vi "Draw Tree.vi"(10 "Sequencing Data":T1) -> (2 "Tree":T1, 3 "2D Picture":picture)   [LabVIEW 2025]
uses:
  Types/Decision Tree.ctl
  Types/Sequencing Tree Node.ctl
  Types/Single Cmd Info.ctl
  <vilib>/picture/picture.llb/imagedata.ctl
panel:
  in  "Outcome Font":T5={"Font Name:"="Bahnschrift", "Size"=15, "Strikeout?"=FALSE, "Italic?"=FALSE, "Underline?"=TRUE, "Outline?"=FALSE, "Shadow?"=FALSE, "Bold?"=TRUE}
  in  "Height Padding":i32=8
  in  "Leaf + Outcome Name Height":i32=38
  in  "Leaf Width":i32=16
  in  "Command Height":i32=32
  in  "Path on Command Branch Height":i32=35
  in  "Default Path Height":i32=15
  in  "Leaf Height":i32=16
  in  "Leaf Circle Radius":i32=8
  in  "pen":T6={"Width"=3, "Style"=enum."Solid"}
  in  "2D Picture":picture
  in  "Column Gap":i32=30
  in  "[user-specified font]":T5={"Font Name:"="Bahnschrift", "Size"=15, "Strikeout?"=FALSE, "Italic?"=FALSE, "Underline?"=FALSE, "Outline?"=FALSE, "Shadow?"=FALSE, "Bold?"=FALSE}
  in  "Width Padding":i32=8
  in  "Row Gap":i32=40
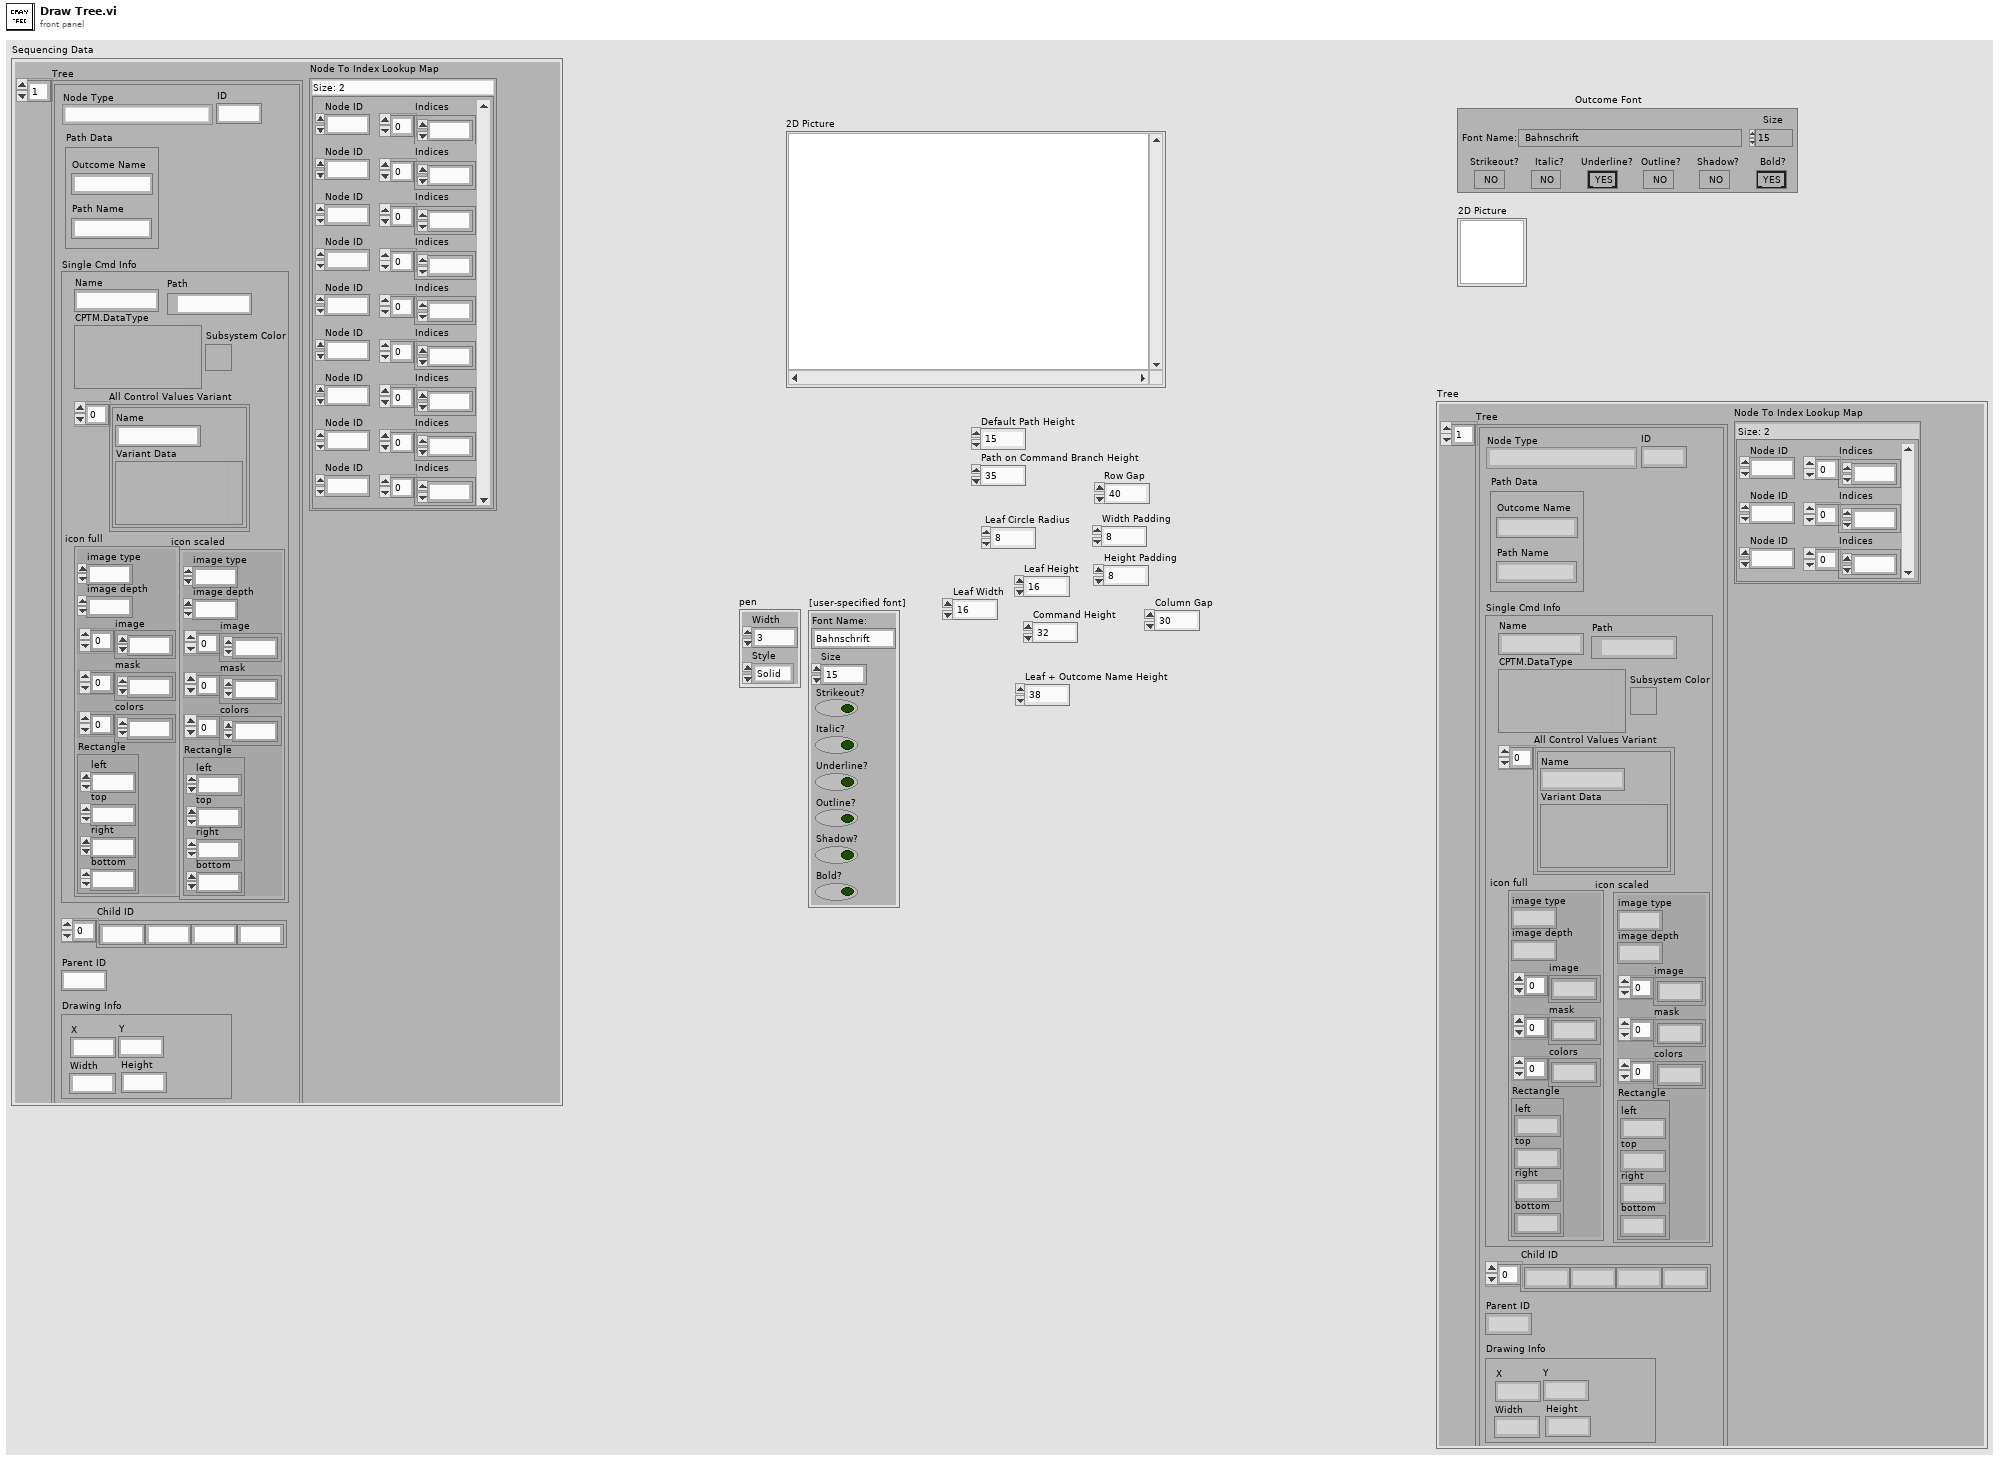
[diagram p1: front panel]
types:
  T1 = typedef "Decision Tree.ctl" = cluster{"Tree":T2[], "Node To Index Lookup Map":map{i16, i16[]}}
  T2 = typedef "Sequencing Tree Node.ctl" = cluster{"Node Type":enum16{"Path", "Command", "Leaf"}, "ID":i16, "Path Data":cluster{"Path Name":string, "Outcome Name":string}, "Single Cmd Info":T3, "Child ID":i32[], "Parent ID":i32, "Drawing Info":cluster{"X":i32, "Y":i32, "Width":i32, "Height":i32}}
  T3 = typedef "Single Cmd Info.ctl" = cluster{"Name":string, "CPTM.DataType":variant, "All Control Values Variant":cluster{"Name":string, "Variant Data":variant}[], "icon full":T4, "icon scaled":T4, "Path":path, "Subsystem Color":u32}
  T4 = typedef "imagedata.ctl" = cluster{"image type":i32, "image depth":i32, "image":u8[], "mask":u8[], "colors":u32[], "Rectangle":cluster{"left":i16, "top":i16, "right":i16, "bottom":i16}}
  T5 = cluster{"Font Name:":string, "Size":i16, "Strikeout?":bool, "Italic?":bool, "Underline?":bool, "Outline?":bool, "Shadow?":bool, "Bold?":bool}
  T6 = cluster{"Width":i16, "Style":enum32{"Solid", "Dash", "Dot", "DashDot", "DashDotDot"}}
  T7 = cluster{"X":i32, "Y":i32, "Width":i32, "Height":i32}
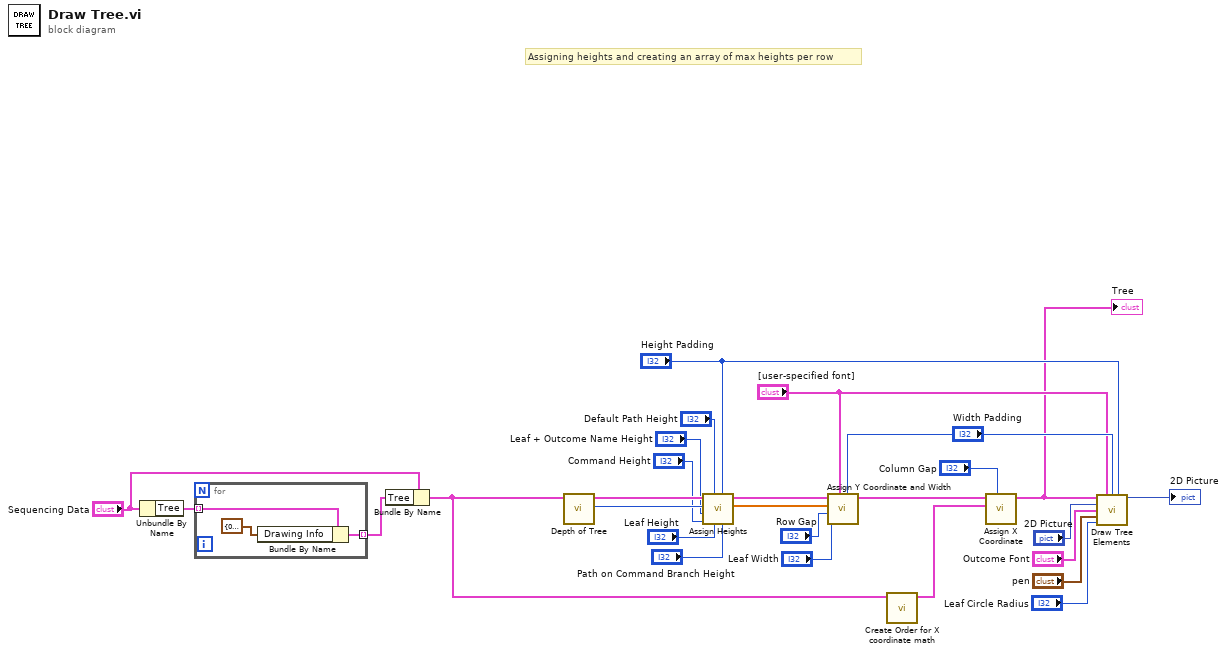
[diagram p0: block diagram]
diagram:
  # "Assigning heights and creating an array of max heights per row"
  n1 = Unbundle By Name("Sequencing Data") -> ("Tree"=w4:T2[])
  n2 = for {
    tunnel: w4 -> [w30] mode=indexing
    tunnel: [w28] -> w3 mode=indexing
    n3 = Bundle By Name(cluster=w30, "Drawing Info"=T7 {"X"=0, "Y"=0, "Width"=0, "Height"=0}) -> (w28:T2)
  }
  n4 = Bundle By Name(cluster="Sequencing Data", "Tree"=w3) -> (w1:T1)
  n5 = call "Depth of Tree.vi"("Tree in"=w1) -> ("Depth"=w24:i32, "Tree with Depths"=w27:T1)  [unwired: 9 in]
  n6 = call "Assign Heights.vi"("Path on Command Branch Height"="Path on Command Branch Height", "Height Padding"="Height Padding", "Leaf Height"="Leaf Height", "Default Path Height"="Default Path Height", "Command Height"="Command Height", "Leaf + Outcome Name Height"="Leaf + Outcome Name Height", "Depth"=w24, "Tree with Depths in"=w27) -> ("Max Height per Row"=w16:dbl[], "Tree with Heights Out"=w17:T1)  [unwired: 2 in]
  n7 = call "Assign Y Coordinate and Width.vi"("Width Padding"="Width Padding", "[user-specified font]"="[user-specified font]", "Leaf Width"="Leaf Width", "Row Gap"="Row Gap", "Max Height per Row"=w16, "Tree with Heights in"=w17) -> ("Decision Tree Out"=w26:T1)  [unwired: 5 in]
  n8 = call "Create Order for X coordinate math.vi"("Tree"=w1) -> ("Array"=w25:T2[])  [unwired: 10 in]
  n9 = call "Assign X Coordinate.vi"("Column Gap"="Column Gap", "Order"=w25, "Decision Tree Out in"=w26) -> ("Decision Tree Out out"=w5:T1)  [unwired: 8 in]
  "Tree" <- w5
  n10 = call "Draw Tree Elements.vi"("Decision Tree In"=w5, "[user-specified font]"="[user-specified font]", "Width Padding"="Width Padding", "Height Padding"="Height Padding", "2D Picture in"="2D Picture", "Outcome Font"="Outcome Font", "pen"="pen", "Leaf Circle Radius"="Leaf Circle Radius") -> ("2D Picture out"=→"2D Picture":picture)  [unwired: 7 in]
